vi "Set Map Bearing.vi"(8 "Error In":errorcluster, 11 "Bearing (0 - 359)":sgl) -> (0 "error out":errorcluster)   [LabVIEW 2014]
uses:
  C:/Robotic Systems/Products/AgFalcon/Software/Ground Station/Data/Mapping DLL/GMap.NET.WindowsForms.dll
  Data/Mapping DLL/GMap.NET.WindowsForms.dll
  Settings File/FGVs/Map Rotation/Methods/Get Map Rotation.vi
  Reference/SubVI/GMap DLL Refernce.vi
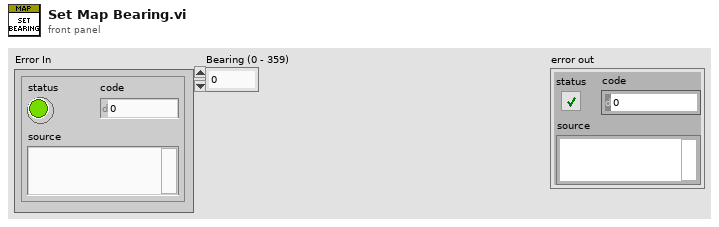
[diagram p1: front panel]
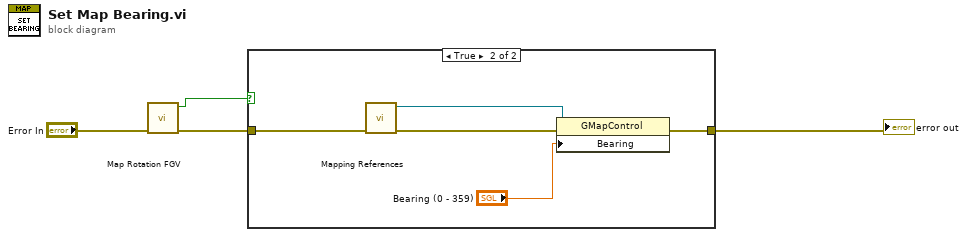
[diagram p0: block diagram]
diagram:
  n1 = call-poly "Map Rotation FGV.vi"("Error In"="Error In") -> ("Error Out"=w2:errorcluster, "Map Rotation On? Out"=w1:bool)  [unwired: 9 in]
  n2 = case shown="True" w1 {
    tunnel: w2 -> [w5 w10]
    tunnel: [w5 w6] -> w4
    frame False {
    }
    frame True {
      n3 = call-poly "Mapping References.vi"("Error In"=w10) -> ("Error Out"=w7:errorcluster, "GMap DLL Reference"=w9:refnum<k24>)  [unwired: 9 in]
      n4 = property class="GMapControl"(reference=w9, error in=w7, "Bearing"="Bearing (0 - 359)") -> (error out=w6:errorcluster)  [unwired: 1 out]
    }
  }
  "error out" <- w4
